vi "Init.vi"(8 "error in (no error)":errorcluster, 10 "Params":variant, 11 "NI SMU in":refnum<class "NI SMU.lvclass">) -> (0 "error out":errorcluster, 3 "NI SMU out":refnum<class "NI SMU.lvclass">)   [LabVIEW 2020, in "NI SMU.lvlib" / "NI SMU.lvclass"]
uses:
  NI SMU.lvclass
  NI SMU.lvclass/NI SMU.ctl
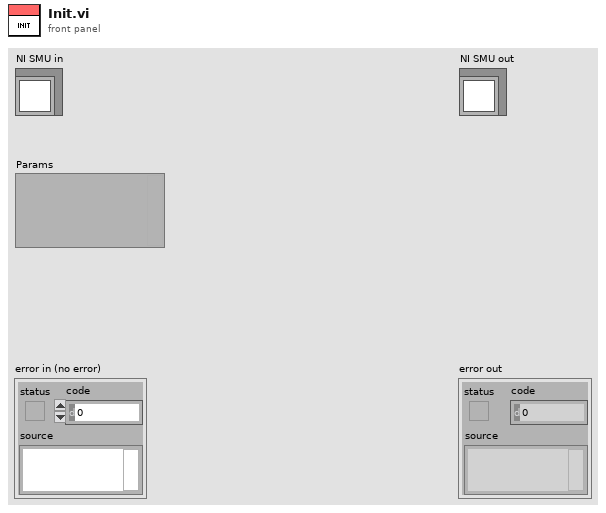
[diagram p1: front panel]
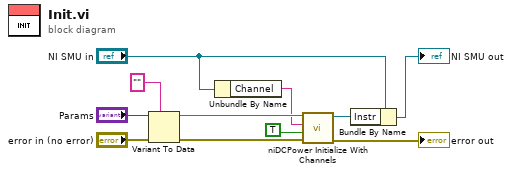
[diagram p0: block diagram]
diagram:
  n1 = Variant To Data(error in="error in (no error)", type="", Variant="Params") -> (data=w7:string, error out=w10:errorcluster)
  n2 = Unbundle By Name("NI SMU in") -> ("Channel"=w2:string)
  n3 = call <instrlib>:"niDCPower Initialize With Channels.vi"("error in (no error)"=w10, "reset (false)"=TRUE, "channels"=w2, "resource name"=w7) -> ("error out"=→"error out":errorcluster, "instrument handle out"=w4:refnum<k15>)  [unwired: 6 in]
  n4 = Bundle By Name(cluster="NI SMU in", "Instr"=w4) -> (→"NI SMU out":refnum<class "NI SMU.lvclass">)
